vi "CSM - Status Change Event.vi"(8 "Error in":errorcluster caption="Error in (no error)", 11 "Name(\"\" to use uuid) in":string) -> (0 "Error out":errorcluster, 3 "Status Change Event":refnum<user-event>)   [LabVIEW 2020, in "Communicable State Machine.lvlib"]
doc: "Obtain CSM Global Log Event Reference.\n- <b>Error in</b>: Error cluster\n- <b>CSM Global Log Event</b>: User event reference for CSM global log.\n- <b>Error out</b>: Error cluster\n\n<b>Inputs:</b>\n - <b>Error in</b>:\n - <b>Name(\"\" to use uuid) in</b>:\n\n<b>Outputs:</b>\n - <b>Error out</b>:\n - <b>Status Change Event</b>:"
uses:
  Communicable State Machine.lvlib
  _CSM Status Change Event Data.ctl
  _CSMOFGVOPER.ctl
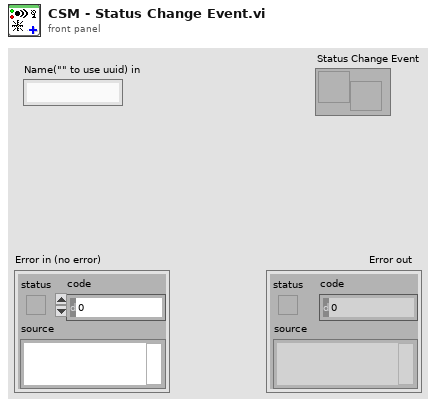
[diagram p1: front panel]
types:
  T1 = typedef "Communicable State Machine.lvlib/_CSMOFGVOPER.ctl" = enum16{"Create If not Exist", "Get By Name", "List", "Check If Name Exists", "Release", "Module Status", "Create Status Event Handler", "Destroy Status Event Handler"}
  T2 = typedef "Communicable State Machine.lvlib/_CSMObj.ctl" = cluster{"Requested Name":string, "Module Name":string, "Mode":T3, "Queue":refnum<class "Priority Queue.lvclass">, "CSM-Data":refnum<data-value>, "User Event":refnum<user-event>, "Status Change Event":refnum<user-event>, "Allowed Messages":string[], "Mode-Data":refnum<data-value>, "Group Name":string, "Exit Event":refnum<user-event>}
  T3 = typedef "Communicable State Machine.lvlib/_CSM_MODE.ctl" = enum16{"Not Exist", "Stand Alone", "CSM", "Worker Agent", "Worker", "Chain", "Chain Node"}
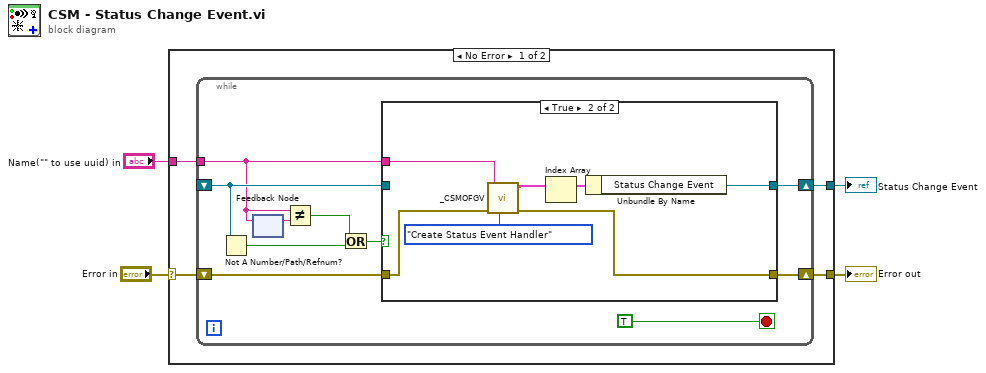
[diagram p0: block diagram]
diagram:
  n1 = case shown="No Error" "Error in" {
    selector: "Error in" -> [w7 w28]
    tunnel: [w8 _] -> w2
    tunnel: [w6 w28] -> w3
    tunnel: "Name(\"\" to use uuid) in" -> [w5 _]
    frame No Error {
      n2 = while {
        shift-right: [w16] -> w6
        shift-left: w7 -> [w17]
        shift-right: [w18] -> w8
        shift-left: _ -> [w14]
        tunnel: w5 -> [w12]
        stop <- TRUE stop-if-true
        n3 = Not A Number/Path/Refnum?(number/path/refnum=w14) -> (NaN/Path/Refnum?=w10:bool)
        n4 = feedback-in #1(w12) -> ()
        n5 = feedback #1() -> (w11:string)  [unwired: 1 in]
        n6 = Not Equal?(x=w12, y=w11) -> (x != y?=w9:bool)
        n7 = Or(x=w9, y=w10) -> (x .or. y?=w13:bool)
        n8 = case shown="True" w13 {
          tunnel: [w20 w22] -> w18
          tunnel: w17 -> [w19 w25]
          tunnel: [w19 w26] -> w16
          tunnel: w14 -> [w20 _]
          tunnel: w12 -> [_ w21]
          frame False {
          }
          frame True {
            n9 = call "_CSMOFGV.vi"("Operation"=_CSMOFGVOPER."Create Status Event Handler", "Error in"=w25, "Name(\"\" to use uuid) in"=w21) -> ("Error out"=w26:errorcluster, "Array"=w24:T2[])  [unwired: 6 in, 1 out]
            n10 = Index Array(array=w24) -> (element=w23:T2)  [unwired: 1 in]
            n11 = Unbundle By Name(w23) -> ("Status Change Event"=w22:refnum<user-event>)
          }
        }
      }
    }
    frame Error {
    }
  }
  "Error out" <- w3
  "Status Change Event" <- w2
